vi "Program_Create.vi"(8 "Error In":errorcluster, 11 "reference in":refnum<class "Program.lvclass">) -> (0 "Error Out":errorcluster, 3 "reference out":refnum<class "Program.lvclass">)   [LabVIEW 2020, in "Program.lvclass"]
uses:
  Program.lvclass
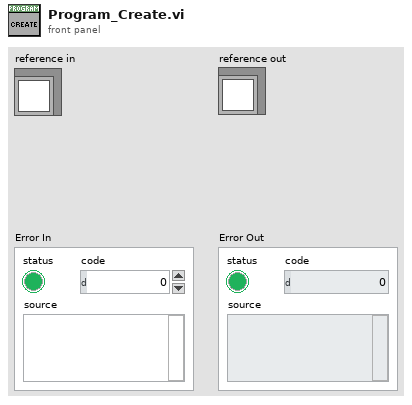
[diagram p1: front panel]
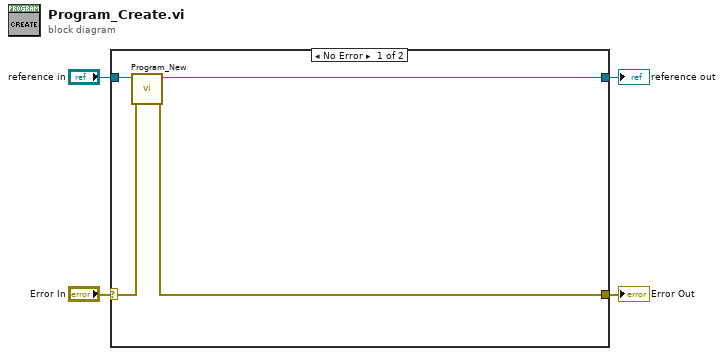
[diagram p0: block diagram]
diagram:
  n1 = case shown="No Error" "Error In" {
    selector: "Error In" -> [w7 w10]
    tunnel: [w5 w10] -> w3
    tunnel: "reference in" -> [w8 w9]
    tunnel: [w6 w9] -> w1
    frame No Error {
      n2 = call "Program_New.vi"("error in (no error)"=w7, "reference in"=w8) -> ("error out"=w5:errorcluster, "reference out"=w6:refnum<class "Program.lvclass">)  [unwired: 6 in, 2 out]
    }
    frame Error {
      # "VI-TechBaseTemplate_Simple_4x4x4"
    }
  }
  "Error Out" <- w3
  "reference out" <- w1
